vi "Cleanup.vi"(11 "MySquare in":refnum<class "MySquare.lvclass">) -> ()   [LabVIEW 2020, in "Galaxy.lvlib" / "MySquare.lvclass"]
uses:
  MySquare.lvclass
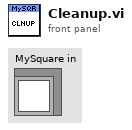
[diagram p1: front panel]
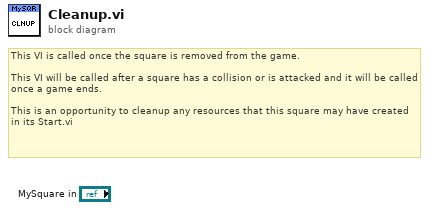
[diagram p0: block diagram]
diagram:
  # "This VI is called once the square is removed from the game.\n\nThis VI will be called after a square has a collision or is attacked and it will be called once a game ends.\n\nThis is an opportunity to cleanup any resources that this square may have created in its Start.vi"
